vi "BuildMenu.vi"(0 "XRef":T7, 1 "MenuRef":T6, 2 "Point":T4, 3 "Menu Type":T3, 4 "State In":T2) -> (14 "Fatal Error Out":T1)   [LabVIEW 2015, in "Set Object Parameters.xnode"]
uses:
  Set Object Parameters.xnode
  <vilib>/XNodeSupport/XNodeXNodeRef.ctl
  <vilib>/XNodeSupport/XNodeMenuRef.ctl
  <vilib>/XNodeSupport/XNodePoint.ctl
  <vilib>/XNodeSupport/XNodeInt.ctl
  <vilib>/XNodeSupport/XNodeMenuType.ctl
  State.ctl
  <vilib>/XNodeSupport/XNodeErrorCluster.ctl
  dimensions.vi
  <vilib>/XNodeSupport/NI_XNodeSupport.lvlib
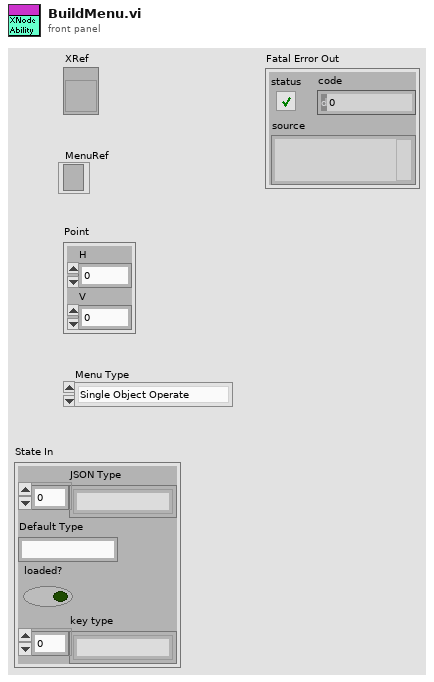
[diagram p1: front panel]
types:
  T1 = typedef "NI_XNodeSupport.lvlib/XNodeErrorCluster.ctl" = errorcluster
  T2 = typedef "Set Object Parameters.xnode/State.ctl" = cluster{"JSON Type":string[], "Default Type":string, "loaded?":bool, "key type":string[]}
  T3 = typedef "NI_XNodeSupport.lvlib/XNodeMenuType.ctl" = enum32{"Single Object Operate", "Single Object Popup", "Multi Object Popup Master", "Multi Object Popup Other"}
  T4 = typedef "NI_XNodeSupport.lvlib/XNodePoint.ctl" = cluster{"H":T5, "V":T5}
  T5 = typedef "NI_XNodeSupport.lvlib/XNodeInt.ctl" = i32
  T6 = typedef "NI_XNodeSupport.lvlib/XNodeMenuRef.ctl" = refnum<k9>
  T7 = typedef "NI_XNodeSupport.lvlib/XNodeXNodeRef.ctl" = refnum<vi>
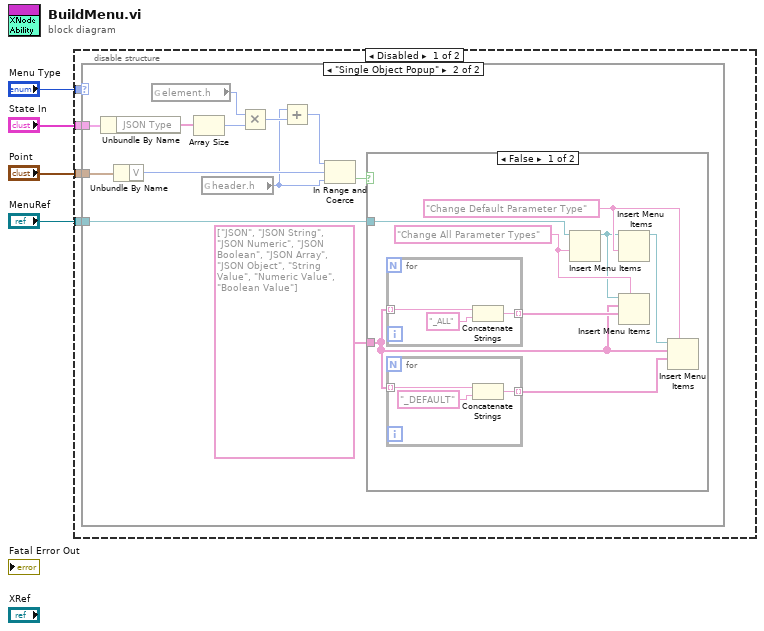
[diagram p0: block diagram]
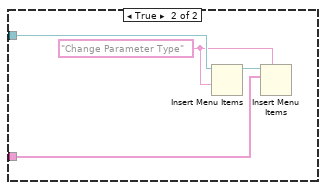
[diagram p3: hidden frame]
diagram:
  n1 = disable-structure shown="Disabled" {
    disable-tunnel: "MenuRef" -> [w8 _]
    disable-tunnel: "Point" -> [w7 _]
    disable-tunnel: "State In" -> [w6 _]
    disable-tunnel: "Menu Type" -> [w5 _]
    frame Disabled {
      n2 = case shown="\"Single Object Popup\"" w5 {
        tunnel: w8 -> [_ w20]
        tunnel: w7 -> [_ w19]
        tunnel: w6 -> [_ w18]
        frame "Single Object Operate", Default {
        }
        frame "Single Object Popup" {
          n3 = Unbundle By Name(w18) -> ("JSON Type"=w11:string[])
          n4 = Unbundle By Name(w19) -> ("V"=w14:T5)
          n5 = global read "dimensions.vi" "element.h"() -> (w17:i16)
          n6 = Array Size(array=w11) -> (size(s)=w10:i32)
          n7 = global read "dimensions.vi" "header.h"() -> (w12:i16)
          n8 = Multiply(x=w17, y=w10) -> (x*y=w16:i32)
          n9 = Add(x=w12, y=w16) -> (x+y=w13:i32)
          n10 = In Range and Coerce(upper limit=w13, x=w14, lower limit=w12) -> (In Range?=w15:bool)  [unwired: 1 out]
          n11 = case shown="False" w15 {
            tunnel: w20 -> [w28 w38]
            tunnel: string[] ["JSON", "JSON String", "JSON Numeric", "JSON Boolean", "JSON Array", "JSON Object", "String Value", "Numeric Value", "Boolean Value"] ("item names") -> [w21 w35]
            frame False {
              w24 = "Change Default Parameter Type" ("menu tag")
              w27 = "Change All Parameter Types" ("menu tag")
              n12 = for {
                tunnel: w21 -> [w34] mode=indexing
                tunnel: [w32] -> w26 mode=indexing
                n13 = Concatenate Strings(w34, "_ALL" ("string")) -> (w32:string)
              }
              n14 = for {
                tunnel: w21 -> [w31] mode=indexing
                tunnel: [w29] -> w25 mode=indexing
                n15 = Concatenate Strings(w31, "_DEFAULT" ("string")) -> (w29:string)
              }
              n16 = Insert Menu Items(7:w27, 9:w28) -> (3:w22:refnum<k9>)  [unwired: 4 in, 2 out]
              n17 = Insert Menu Items(7:w24, 9:w22) -> (3:w23:refnum<k9>)  [unwired: 4 in, 2 out]
              n18 = Insert Menu Items(5:w27, 7:w26, 8:w21, 9:w22) -> ()  [unwired: 2 in, 3 out]
              n19 = Insert Menu Items(5:w24, 7:w25, 8:w21, 9:w23) -> ()  [unwired: 2 in, 3 out]
            }
            frame True {
              w36 = "Change Parameter Type"
              n20 = Insert Menu Items(7:w36, 9:w38) -> (3:w37:refnum<k9>)  [unwired: 4 in, 2 out]
              n21 = Insert Menu Items(5:w36, 8:w35, 9:w37) -> ()  [unwired: 3 in, 3 out]
            }
          }
        }
      }
    }
    frame Enabled {
    }
  }
